vi "G#Debugger_GetRefToCache.vi"(0 "MethodVIref":refnum<vi>, 5 "error in (no error)":errorcluster) -> (15 "cached object out":refnum<class "G#Object.lvclass">, 16 "valid":bool, 19 "error out":errorcluster)   [LabVIEW 2017, in "G#Debugger.lvlib"]
uses:
  G#Debugger.lvlib
  G#Object/G#Object.lvclass
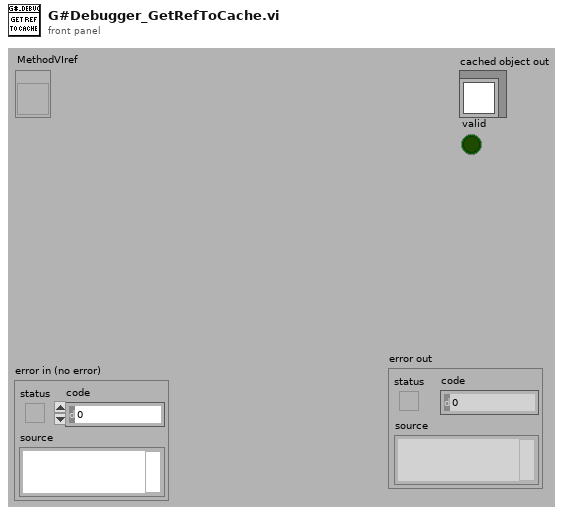
[diagram p1: front panel]
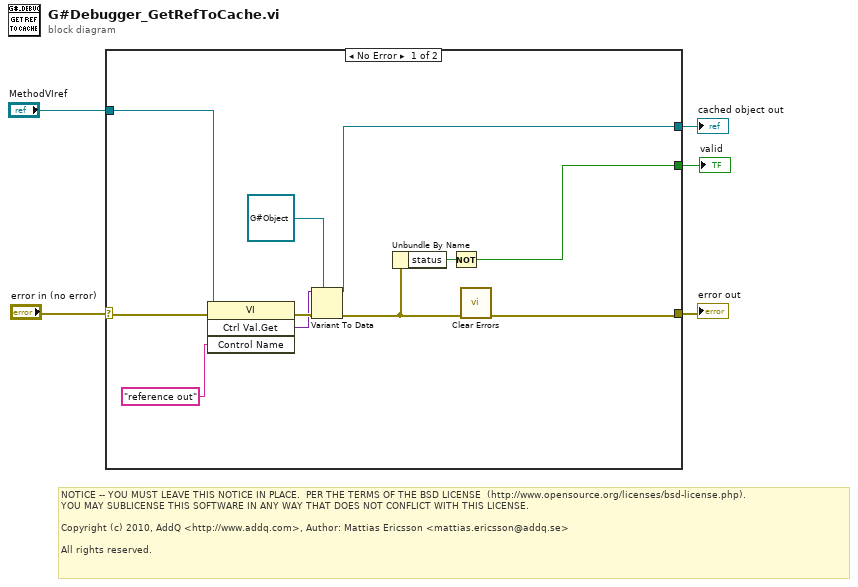
[diagram p0: block diagram]
diagram:
  # "NOTICE -- YOU MUST LEAVE THIS NOTICE IN PLACE.  PER THE TERMS OF THE BSD LICENSE  (http://www.opensource.org/licenses/bsd-license.php).\nYOU MAY SUBLICENSE THIS SOFTWARE IN ANY WAY THAT DOES NOT CONFLICT WITH THIS LICENSE.\n\nCopyright (c) 2010, AddQ <http://www.addq.com>, Author: Mattias Ericsson <mattias.ericsson@addq.se>\n\nAll rights reserved."
  n1 = case shown="No Error" "error in (no error)" {
    selector: "error in (no error)" -> [w12 w17]
    tunnel: [w6 w17] -> w4
    tunnel: "MethodVIref" -> [w16 _]
    tunnel: [w8 _] -> w2
    tunnel: [w7 _] -> w1
    frame No Error {
      n2 = invoke class="VI" method="Ctrl Val.Get"(reference=w16, error in=w12, "Control Name"="reference out") -> (error out=w14:errorcluster, "Get Control Value Variant"=w13:variant)  [unwired: 1 in, 2 out]
      n3 = Variant To Data(error in=w14, type=refnum<class "G#Object.lvclass"> refnum ("G#Object.lvclass"), Variant=w13) -> (data=w8:refnum<class "G#Object.lvclass">, error out=w10:errorcluster)
      n4 = Unbundle By Name(w10) -> ("status"=w9:bool)
      n5 = Not(x=w9) -> (.not. x?=w7:bool)
      n6 = call <vilib>:"Clear Errors.vi"("error in (no error)"=w10) -> ("error out"=w6:errorcluster)  [unwired: 5 in, 1 out]
    }
    frame Error {
    }
  }
  "error out" <- w4
  "cached object out" <- w2
  "valid" <- w1
